vi "Questionable Event Enable.vi"(0 "VISA resource name":refnum<visa-resource-name>, 5 "Questionable Event Enable":T1, 11 "error in (no error)":errorcluster) -> (4 "VISA resource name out":refnum<visa-resource-name>, 15 "error out":errorcluster)   [LabVIEW 2018, in "XP Power PLS600.lvlib"]
doc: "Sets the value of the Questionable Enable register. This register is a mask for enabling specific bits from the Questionable Event register to set the questionable summary (QUES) bit of the Status Byte register. This bit (bit 3) is the logical OR of all the Questionable Event register bits that are enabled by the Questionable Status Enable register.\n\nThe Operation Event Enable consists of the following 16 bits:\n\nBit 0: Summary of Voltage\nBit 1: Summary of Current\nBit 2: Summary of Time \nBit 3: Summary of Power\nBit 4: Summary of Temperature\nBit 5: Summary of Frequency \nBit 6: Summary of Phase\nBit 7: Summary of Modulation\nBit 8: Summary of Calibration\nBit 9: Summary of Hardware\nBit 10: Watchdog Error\nBit 11: Self-Test Error\nBit 12: Regulation Loss Error\nBit 13: Instrument Summary\nBit 14: Command Warning\nBit 15: Reserved"
uses:
  XP Power PLS600.lvlib
panel:
  # "Bit 0: Summary of Voltage\nBit 1: Summary of Current\nBit 2: Summary of Time\t\nBit 3: Summary of Power\nBit 4:\tSummary of Temperature\nBit 5: Summary of Frequency\t\nBit 6: Summary of Phase\nBit 7: Summary of Modulation\nBit 8: Summary of Calibration\nBit 9: Summary of Hardware\nBit 10: Watchdog Error\nBit 11: Self-Test Error\nBit 12: Regulation Loss Error\nBit 13: Instrument Summary\nBit 14: Command Warning\nBit 15: Reserved"
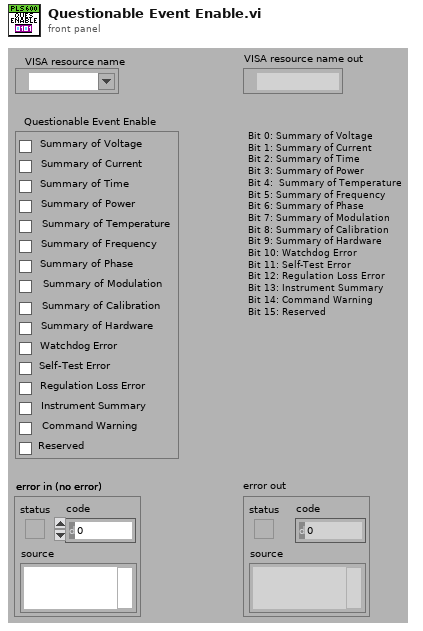
[diagram p1: front panel]
types:
  T1 = cluster{"Summary of Voltage":bool, "Summary of Current":bool, "Summary of Time":bool, "Summary of Power":bool, "Summary of Temperature":bool, "Summary of Frequency":bool, "Summary of Phase":bool, "Summary of Modulation":bool, "Summary of Calibration":bool, "Summary of Hardware":bool, "Watchdog Error":bool, "Self-Test Error":bool, "Regulation Loss Error":bool, "Instrument Summary":bool, "Command Warning":bool, "Reserved":bool}
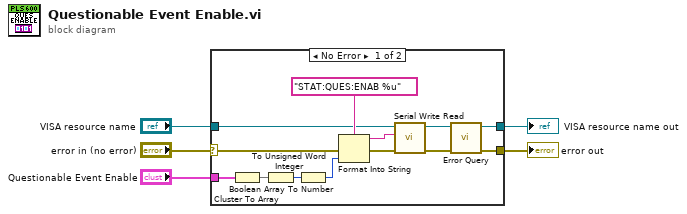
[diagram p0: block diagram]
diagram:
  n1 = case shown="No Error" "error in (no error)" {
    selector: "error in (no error)" -> [w18 w20]
    tunnel: "VISA resource name" -> [w11 w19]
    tunnel: [w6 w19] -> w5
    tunnel: [w7 w20] -> w4
    tunnel: "Questionable Event Enable" -> [w15 _]
    frame No Error {
      n2 = Cluster To Array(cluster=w15) -> (array=w16:bool[])
      n3 = Boolean Array To Number(Boolean array=w16) -> (number=w14:u32)
      n4 = To Unsigned Word Integer(number=w14) -> (unsigned 16bit integer=w13:u16)
      n5 = Format Into String(format string="STAT:QUES:ENAB %u" ("Command to Send"), error in=w18, w13) -> (resulting string=w10:string, error out=w9:errorcluster)  [unwired: 1 in]
      n6 = call "Serial Write Read.vi"("error in (no error)"=w9, "Write Buffer"=w10, "VISA resource name"=w11) -> ("error out"=w8:errorcluster, "VISA resource name out"=w12:refnum<visa-resource-name>)  [unwired: 6 in, 1 out]
      n7 = call "Error Query.vi"("error in (no error)"=w8, "VISA resource name"=w12) -> ("error out"=w7:errorcluster, "VISA resource name out"=w6:refnum<visa-resource-name>)  [unwired: 6 in, 2 out]
    }
    frame Error {
    }
  }
  "error out" <- w4
  "VISA resource name out" <- w5
